vi "CreateEAN-13Checksum.vi"(8 "error in (no error)":errorcluster, 10 "String":string, 11 "EAN-13 in":refnum<class "EAN-13.lvclass">) -> (0 "error out":errorcluster, 2 "Checksum":string, 3 "EAN-13 out":refnum<class "EAN-13.lvclass">)   [LabVIEW 2013, in "BarCodes.lvlib" / "EAN-13.lvclass"]
doc: "Creates a checksum for EAN-13 and returns it as a character to add to the input string"
uses:
  EAN-13.lvclass
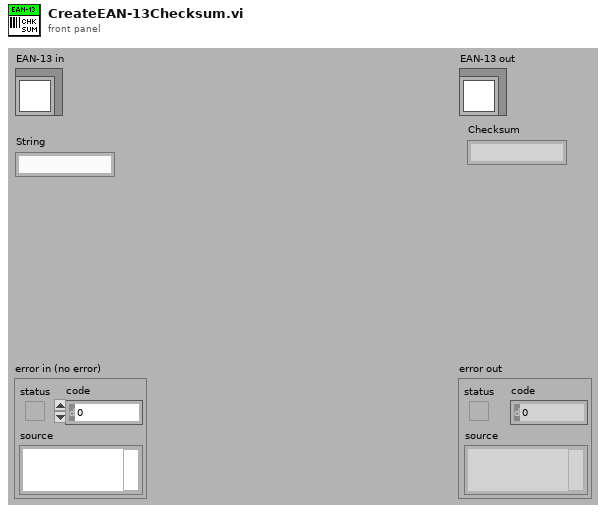
[diagram p1: front panel]
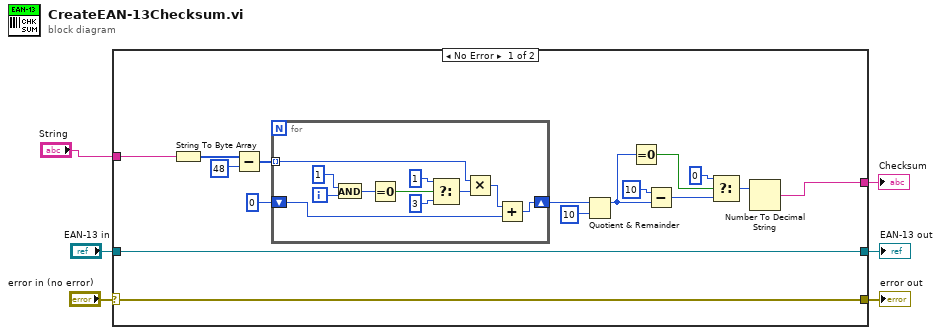
[diagram p0: block diagram]
diagram:
  n1 = case shown="No Error" "error in (no error)" {
    selector: "error in (no error)" -> [w21 w35]
    tunnel: [w21 w35] -> w5
    tunnel: [w22 w34] -> w3
    tunnel: "EAN-13 in" -> [w22 w34]
    tunnel: [w8 _] -> w2
    tunnel: "String" -> [w7 _]
    frame No Error {
      n2 = String To Byte Array(string=w7) -> (unsigned byte array=w20:u8[])
      n3 = Subtract(x=w20, y=u8 48) -> (x-y=w11:u8[])
      n4 = for {
        tunnel: w11 -> [w31] mode=indexing
        shift-right: [w24] -> w9
        shift-left: 0 -> [w23]
        i -> [w33]
        n5 = And(x=1, y=w33) -> (x .and. y?=w30:i32)
        n6 = Equal To 0?(x=w30) -> (x = 0?=w29:bool)
        n7 = Select(t=1, s=w29, f=3 ("x")) -> (s? t:f=w26:i32)
        n8 = Multiply(x=w31, y=w26) -> (x*y=w25:i32)
        n9 = Add(x=w25, y=w23) -> (x+y=w24:i32)
      }
      n10 = Quotient & Remainder(x=w9, y=u8 10) -> (x-y*floor(x/y)=w14:i32)  [unwired: 1 out]
      n11 = Equal To 0?(x=w14) -> (x = 0?=w17:bool)
      n12 = Subtract(x=u8 10 ("y"), y=w14) -> (x-y=w13:i32)
      n13 = Select(t=u8 0 ("y"), s=w17, f=w13) -> (s? t:f=w12:i32)
      n14 = Number To Decimal String(number=w12) -> (decimal integer string=w8:string)  [unwired: 1 in]
    }
    frame Error {
    }
  }
  "error out" <- w5
  "EAN-13 out" <- w3
  "Checksum" <- w2
